vi "Process Data Motor Read_vel.vi"(11 "에러 입력(에러 없음)":errorcluster) -> (4 "Actual Pos_0":i32, 6 "Actual Vel_0":i32, 8 "Actual Pos_1":i32, 10 "Actual Vel_1":i32, 13 "Actual_Cur_1":i16, 14 "Actual_Cur_0":i16, 15 "에러 출력":errorcluster)   [LabVIEW 2019]
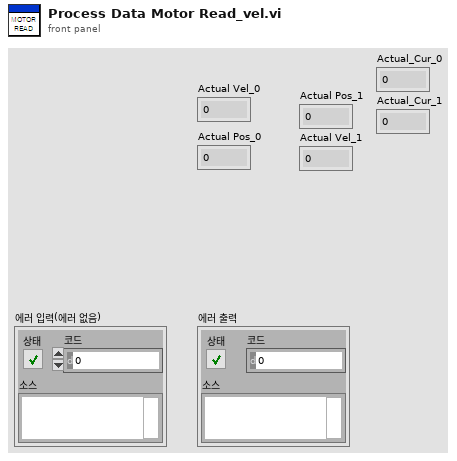
[diagram p1: front panel]
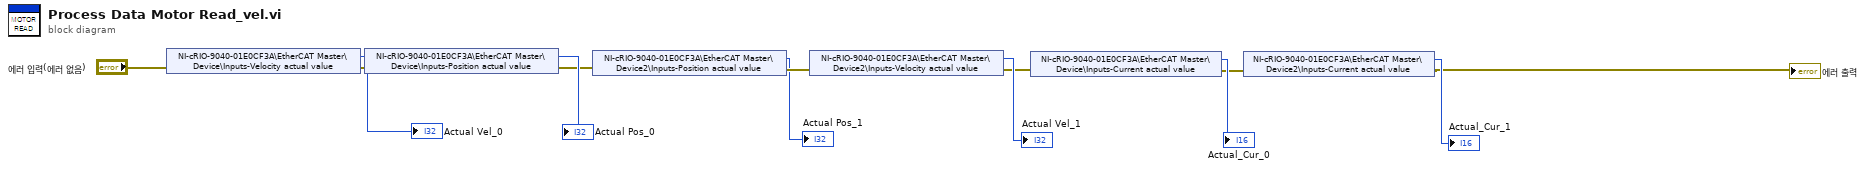
[diagram p0: block diagram]
diagram:
  n1 = shared-variable "NI-cRIO-9040-01E0CF3A\\EtherCAT Master\\Device\\Inputs-Velocity actual value"(error in="에러 입력(에러 없음)") -> (→"Actual Vel_0":i32, error out=w13:errorcluster)
  n2 = shared-variable "NI-cRIO-9040-01E0CF3A\\EtherCAT Master\\Device\\Inputs-Position actual value"(error in=w13) -> (→"Actual Pos_0":i32, error out=w9:errorcluster)
  n3 = shared-variable "NI-cRIO-9040-01E0CF3A\\EtherCAT Master\\Device2\\Inputs-Position actual value"(error in=w9) -> (→"Actual Pos_1":i32, error out=w8:errorcluster)
  n4 = shared-variable "NI-cRIO-9040-01E0CF3A\\EtherCAT Master\\Device2\\Inputs-Velocity actual value"(error in=w8) -> (→"Actual Vel_1":i32, error out=w3:errorcluster)
  n5 = shared-variable "NI-cRIO-9040-01E0CF3A\\EtherCAT Master\\Device\\Inputs-Current actual value"(error in=w3) -> (→"Actual_Cur_0":i16, error out=w2:errorcluster)
  n6 = shared-variable "NI-cRIO-9040-01E0CF3A\\EtherCAT Master\\Device2\\Inputs-Current actual value"(error in=w2) -> (→"Actual_Cur_1":i16, error out=→"에러 출력":errorcluster)
